vi "step_state.vi"(0 "state in":T1={"State"=enum."sense", "Maze"=[[FALSE, FALSE, FALSE, FALSE, FALSE, FALSE, FALSE, FALSE, FALSE], [FALSE, FALSE, TRUE, FALSE, FALSE, TRUE, TRUE, TRUE, FALSE], [FALSE, FALSE, TRUE, TRUE, TRUE, TRUE, FALSE, FALSE, FALSE], [FALSE, FALSE, TRUE, FALSE, FALSE, TRUE, FALSE, FALSE, FALSE], [TRUE, TRUE, TRUE, FALSE, FALSE, TRUE, FALSE, TRUE, TRUE], [FALSE, FALSE, FALSE, TRUE, TRUE, TRUE, FALSE, TRUE, FALSE], [FALSE, FALSE, FALSE, FALSE, FALSE, TRUE, TRUE, TRUE, FALSE], [FALSE, FALSE, FALSE, FALSE, FALSE, FALSE, FALSE, FALSE, FALSE], [FALSE, FALSE, FALSE, FALSE, FALSE, FALSE, FALSE, FALSE, FALSE]], "Runner Row"=0, "Runner Column"=0, "Runner Direction"=enum."east", "Sense"={"wall in front"=FALSE, "wall to left"=FALSE, "wall to right"=FALSE, "wall behind"=FALSE, "exit column"=FALSE}, "Hand"=enum."Left-handed"}) -> (4 "state out":T1={"State"=enum."sense", "Maze"=[[FALSE, FALSE, FALSE, FALSE, FALSE, FALSE, FALSE, FALSE, FALSE], [FALSE, FALSE, TRUE, FALSE, FALSE, TRUE, TRUE, TRUE, FALSE], [FALSE, FALSE, TRUE, TRUE, TRUE, TRUE, FALSE, FALSE, FALSE], [FALSE, FALSE, TRUE, FALSE, FALSE, TRUE, FALSE, FALSE, FALSE], [TRUE, TRUE, TRUE, FALSE, FALSE, TRUE, FALSE, TRUE, TRUE], [FALSE, FALSE, FALSE, TRUE, TRUE, TRUE, FALSE, TRUE, FALSE], [FALSE, FALSE, FALSE, FALSE, FALSE, TRUE, TRUE, TRUE, FALSE], [FALSE, FALSE, FALSE, FALSE, FALSE, FALSE, FALSE, FALSE, FALSE], [FALSE, FALSE, FALSE, FALSE, FALSE, FALSE, FALSE, FALSE, FALSE]], "Runner Row"=0, "Runner Column"=0, "Runner Direction"=enum."east", "Sense"={"wall in front"=FALSE, "wall to left"=FALSE, "wall to right"=FALSE, "wall behind"=FALSE, "exit column"=FALSE}, "Hand"=enum."Left-handed"})   [LabVIEW 2016]
uses:
  typedefs/state.ctl
  typedefs/action_start.ctl
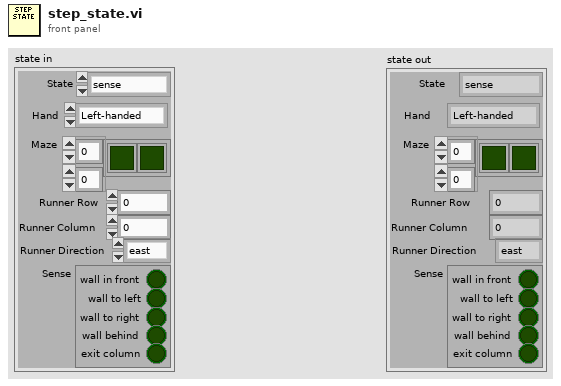
[diagram p1: front panel]
types:
  T1 = typedef "state.ctl" = cluster{"State":T2, "Maze":bool[][], "Runner Row":i32, "Runner Column":i32, "Runner Direction":enum16{"east", "north", "west", "south"}, "Sense":cluster{"wall in front":bool, "wall to left":bool, "wall to right":bool, "wall behind":bool, "exit column":bool}, "Hand":enum16{"Left-handed", "Right-handed"}}
  T2 = typedef "action_start.ctl" = enum16{"sense", "decide", "step", "pivot right", "pivot left", "stop"}
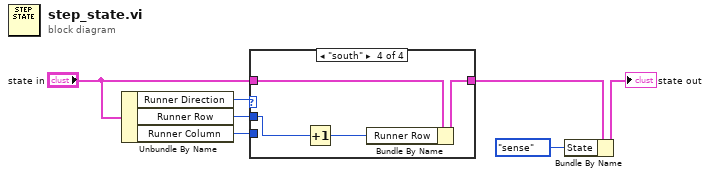
[diagram p0: block diagram]
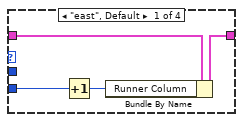
[diagram p2: hidden frame]
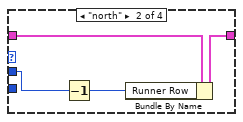
[diagram p3: hidden frame]
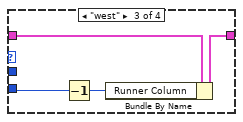
[diagram p4: hidden frame]
diagram:
  n1 = Unbundle By Name("state in") -> ("Runner Direction"=w6:enum16{"east", "north", "west", "south"}, "Runner Row"=w2:i32, "Runner Column"=w5:i32)
  n2 = case shown="\"south\"" w6 {
    tunnel: w5 -> [w11 _ w16 _]
    tunnel: [w9 w12 w17 w20] -> w3
    tunnel: "state in" -> [w8 w13 w18 w21]
    tunnel: w2 -> [_ w14 _ w22]
    frame "east", Default {
      n3 = Increment(x=w11) -> (x+1=w10:i32)
      n4 = Bundle By Name(cluster=w8, "Runner Column"=w10) -> (w9:T1)
    }
    frame "north" {
      n5 = Decrement(x=w14) -> (x-1=w15:i32)
      n6 = Bundle By Name(cluster=w13, "Runner Row"=w15) -> (w12:T1)
    }
    frame "west" {
      n7 = Decrement(x=w16) -> (x-1=w19:i32)
      n8 = Bundle By Name(cluster=w18, "Runner Column"=w19) -> (w17:T1)
    }
    frame "south" {
      n9 = Increment(x=w22) -> (x+1=w23:i32)
      n10 = Bundle By Name(cluster=w21, "Runner Row"=w23) -> (w20:T1)
    }
  }
  n11 = Bundle By Name(cluster=w3, "State"=action_start."sense" ("action start")) -> (→"state out":T1)
